vi "Add Constants Base from array of constants.vi"(8 "error in (no error)":errorcluster, 11 "Constants Array":T1[](array[typedef])) -> (0 "error out":errorcluster)   [LabVIEW 2013]
uses:
  Constants typedef V2.ctl
  Constants Global.vi
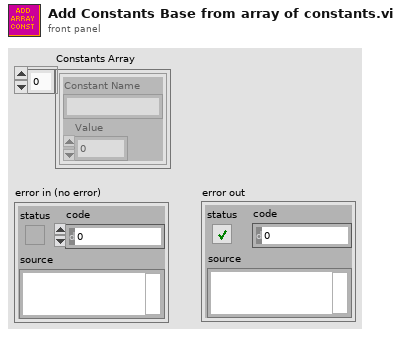
[diagram p1: front panel]
types:
  T1 = typedef "Constants typedef V2.ctl" = cluster{"Constant Name":string, "Value":dbl}
  T2 = typedef "Constants Map typedef.ctl" = cluster{T1[]}[]
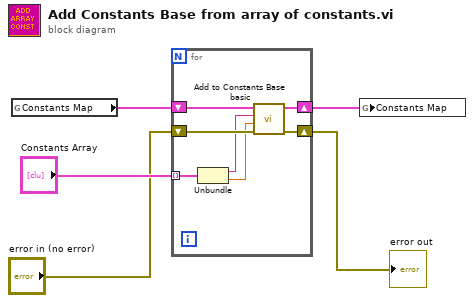
[diagram p0: block diagram]
diagram:
  n1 = global read "Constants Global.vi" "Constants Map"() -> (w4:T2)
  n2 = for {
    tunnel: "Constants Array" -> [w8] mode=indexing
    shift-right: [w12] -> w1
    shift-left: "error in (no error)" -> [w11]
    shift-right: [w10] -> w3
    shift-left: w4 -> [w9]
    n3 = Unbundle(w8) -> ("Constant Name"=w7:string, "Value"=w6:dbl)
    n4 = call "Add to Constants Base basic.vi"("error in (no error)"=w11, "Value"=w6, "Constant Name"=w7, "Constants Map"=w9) -> ("Error out"=w12:errorcluster, "Constants Map out"=w10:T2)  [unwired: 6 in]
  }
  "error out" <- w1
  n5 = global write "Constants Global.vi" "Constants Map"(w3) -> ()
